vi "zad2.vi"() -> ()   [LabVIEW 2018]
uses:
  <vilib>/measure/NI_MABase.lvlib
panel:
  in  "frequency":dbl(slide)=10.0 scale=200.0..2000.0
  out "Waveform Graph 2":i32[][](graph)
  out "Waveform Graph":waveform(dbl)(graph)
  in  "Stop":bool
  in  "amplitude":dbl(slide)=1.0 scale=0.0..10.0
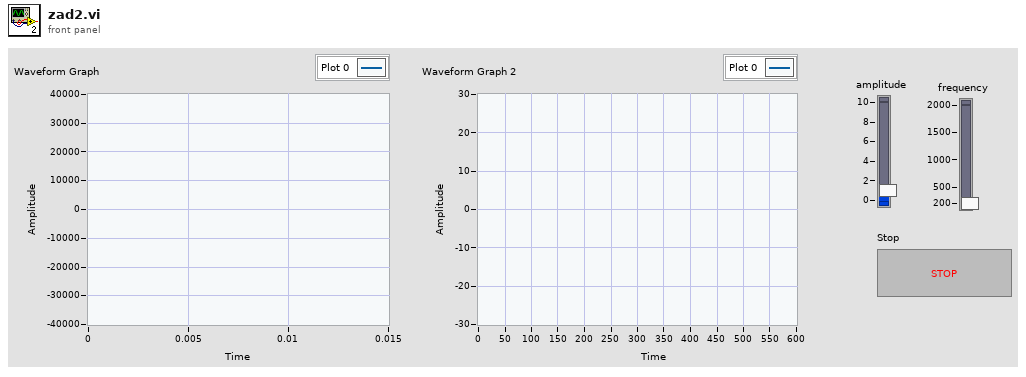
[diagram p1: front panel]
types:
  T1 = cluster{"# buffers":i32, "Buffer size":i32, "unit (ms)":enum16{"time (ms)", "Samples"}}
  T2 = typedef "SoundHandle.ctl" = cluster{"DeviceID":u16, "Samples/buf":u32, "Sampl rate":u32, "Bits/sample":u16, "Channels":u8, "Opened":bool}
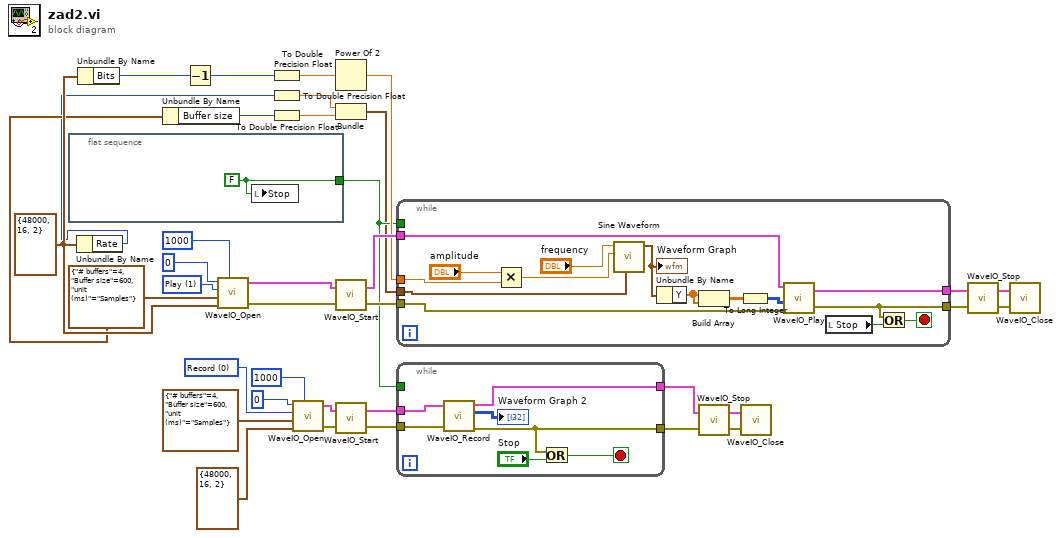
[diagram p0: block diagram]
diagram:
  w14 = u16 0 items=["Record", "Play", "Loopback", "ASIO input", "ASIO output", "Record (WASAPI)", "Play (WASAPI)", "Record Combi", "Play Combi"] ("device type (Record)")
  w29 = cluster{"Rate":i32, "Bits":i32, "Channels":u32} {"Rate"=48000, "Bits"=16, "Channels"=2} ("Format (44kHz, 16Bit, stereo)")
  w28 = T1 {"# buffers"=4, "Buffer size"=600, "unit (ms)"=enum."Samples"} ("Buffer Config")
  w35 = u16 1 items=["Record", "Play", "Loopback", "ASIO input", "ASIO output", "Record (WASAPI)", "Play (WASAPI)", "Record Combi", "Play Combi"] ("device type (Record)")
  n1 = flat-sequence {
    tunnel: [w37] -> w4
    frame #0 {
      w37 = FALSE
      n2 = local write "Stop"(w37) -> ()
    }
  }
  n3 = Unbundle By Name(w29) -> ("Rate"=w27:i32)
  n4 = Unbundle By Name(w29) -> ("Bits"=w31:i32)
  n5 = Unbundle By Name(w28) -> ("Buffer size"=w26:i32)
  n6 = Decrement(x=w31) -> (x-1=w30:i32)
  n7 = call "WaveIO_Open.vi"("idev"=u32 0, "Watchdog timeout (msec) (default=OFF)"=1000, "device type (Record)"=w35, "Buffer Config"=w28, "Format (44kHz, 16Bit, stereo)"=w29) -> ("Sound Handle Out"=w34:T2, "error out"=w33:errorcluster)  [unwired: 2 in]
  n8 = To Double Precision Float(number=w30) -> (double precision float=w25:dbl)
  n9 = To Double Precision Float(number=w27) -> (double precision float=w3:dbl)
  n10 = To Double Precision Float(number=w26) -> (double precision float=w2:dbl)
  n11 = call "WaveIO_Open.vi"("idev"=u32 0, "Watchdog timeout (msec) (default=OFF)"=1000, "device type (Record)"=w14, "Buffer Config"=T1 {"# buffers"=4, "Buffer size"=600, "unit (ms)"=enum."Samples"}, "Format (44kHz, 16Bit, stereo)"=cluster{"Rate":i32, "Bits":i32, "Channels":u32} {"Rate"=48000, "Bits"=16, "Channels"=2}) -> ("Sound Handle Out"=w17:T2, "error out"=w16:errorcluster)  [unwired: 2 in]
  n12 = Power Of 2(x=w25) -> (2^x=w22:dbl)
  n13 = Bundle(w3, w2) -> (w1:cluster{dbl, dbl})  [unwired: 1 in]
  n14 = call "WaveIO_Start.vi"("error in (no error)"=w33, "Handle"=w34) -> ("error out"=w23:errorcluster, "Handle Out"=w24:T2)
  n15 = call "WaveIO_Start.vi"("error in (no error)"=w16, "Handle"=w17) -> ("error out"=w5:errorcluster, "Handle Out"=w6:T2)
  n16 = while {
    tunnel: w24 -> [w50]
    tunnel: w23 -> [w49]
    tunnel: w22 -> [w48]
    tunnel: [w45] -> w21
    tunnel: [w42] -> w20
    tunnel: w4 -> [_]
    tunnel: w1 -> [w40]
    stop <- w43 stop-if-true
    n17 = Multiply(x="amplitude", y=w48) -> (x*y=w46:dbl)
    n18 = call <vilib>:"Sine Waveform.vi"("sampling info"=w40, "amplitude"=w46, "frequency"="frequency") -> ("signal out"=w39:waveform(dbl))  [unwired: 7 in, 1 out]
    "Waveform Graph" <- w39
    n19 = Unbundle By Name(w39) -> ("Y"=w51:dbl[])
    n20 = Build Array(w51, w51) -> (w52:dbl[][])
    n21 = To Long Integer(number=w52) -> (32bit integer=w44:i32[][])
    n22 = call "WaveIO_Play.vi"("error in (no error)"=w49, "data"=w44, "Handle"=w50) -> ("error out"=w42:errorcluster, "Handle Out"=w45:T2)  [unwired: 1 in]
    n23 = local read "Stop"() -> (w41:bool)
    n24 = Or(x=w42, y=w41) -> (x .or. y?=w43:bool)
  }
  n25 = while {
    tunnel: [w59] -> w8
    tunnel: [w54] -> w7
    tunnel: w6 -> [w58]
    tunnel: w5 -> [w57]
    tunnel: w4 -> [_]
    stop <- w56 stop-if-true
    n26 = call "WaveIO_Record.vi"("Handle"=w58, "error in (no error)"=w57) -> ("Handle Out"=w59:T2, "Data"=→"Waveform Graph 2":i32[][], "error out"=w54:errorcluster)  [unwired: 1 in, 2 out]
    n27 = Or(x=w54, y="Stop") -> (x .or. y?=w56:bool)
  }
  n28 = call "WaveIO_Stop.vi"("error in (no error)"=w7, "Handle"=w8) -> ("error out"=w9:errorcluster, "Handle Out"=w10:T2)
  n29 = call "WaveIO_Close.vi"("error in (no error)"=w9, "Handle"=w10) -> ()  [unwired: 2 out]
  n30 = call "WaveIO_Stop.vi"("error in (no error)"=w20, "Handle"=w21) -> ("error out"=w18:errorcluster, "Handle Out"=w19:T2)
  n31 = call "WaveIO_Close.vi"("error in (no error)"=w18, "Handle"=w19) -> ()  [unwired: 2 out]
